vi "sub_error-instr.vi"(7 "instr sel":T1, 11 "error":bool) -> ()   [LabVIEW 2021]
uses:
  ctrl/instr-hw.ctl
  ctrl/ini-rw.ctl
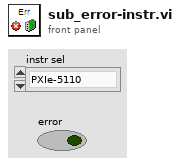
[diagram p1: front panel]
types:
  T1 = typedef "instr-hw.ctl" = enum16{"PXIe-5110", "PXIe-5431", "PXIe-2530", "DS1202"}
  T2 = typedef "ini-rw.ctl" = enum16{"read", "write", "ini"}
  T3 = typedef "error.ctl" = cluster{"PXIe-5110":bool, "PXIe-5431":bool, "PXIe-2530":bool, "DS1202":bool}
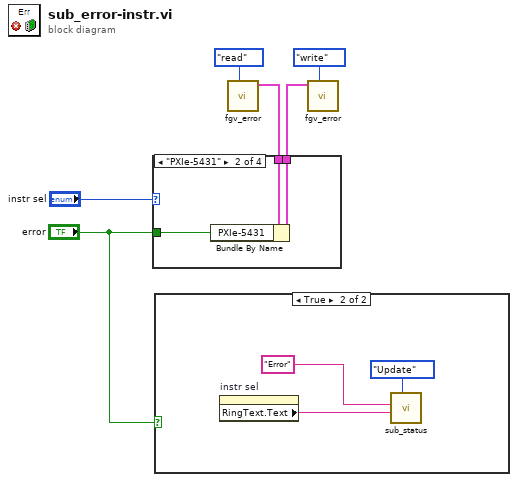
[diagram p0: block diagram]
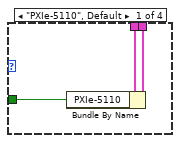
[diagram p3: hidden frame]
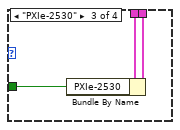
[diagram p4: hidden frame]
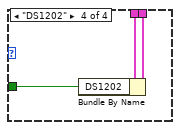
[diagram p5: hidden frame]
diagram:
  n1 = case shown="True" "error" {
    frame False {
    }
    frame True {
      n2 = property on="instr sel" class="Enum (strict)"() -> ("RingText.Text"=w8:string)  [unwired: 2 in, 2 out]
      n3 = call "sub_status.vi"("Mode"=enum16{"Initial", "Update", "Clear"}."Update", "detail"=w8, "title"="Error") -> ()  [unwired: 8 in, 1 out]
    }
  }
  n4 = call "fgv_error.vi"("cmd"=ini-rw."read") -> ("error"=w5:T3)  [unwired: 10 in]
  n5 = case shown="\"PXIe-5431\"" "instr sel" {
    tunnel: [w12 w15 w18 w21] -> w6
    tunnel: w5 -> [w11 w14 w17 w20]
    tunnel: "error" -> [w10 w13 w16 w19]
    frame "PXIe-5110", Default {
      n6 = Bundle By Name(cluster=w11, "PXIe-5110"=w10) -> (w12:T3)
    }
    frame "PXIe-5431" {
      n7 = Bundle By Name(cluster=w14, "PXIe-5431"=w13) -> (w15:T3)
    }
    frame "PXIe-2530" {
      n8 = Bundle By Name(cluster=w17, "PXIe-2530"=w16) -> (w18:T3)
    }
    frame "DS1202" {
      n9 = Bundle By Name(cluster=w20, "DS1202"=w19) -> (w21:T3)
    }
  }
  n10 = call "fgv_error.vi"("cmd"=ini-rw."write", "error 2"=w6) -> ()  [unwired: 9 in, 1 out]
